vi "Send.vi"(5 "Record Topic Name?":bool, 7 "Message Priority":T1, 8 "error in (no error)":errorcluster, 9 "Timeout":i32, 10 "Message":refnum<class "Message Interface.lvclass">, 11 "Message Transport Queue in":refnum<class "Message Transport Queue.lvclass">) -> (0 "error out":errorcluster, 2 "Timed Out?":bool, 3 "Message Transport Queue out":refnum<class "Message Transport Queue.lvclass">)   [LabVIEW 2016, in "Stream Mediator.lvlib" / "Message Transport Queue.lvclass"]
doc: "--\nCopyright © 2017 Composed SystemsI All rights reserved.\n\nAuthor: Jon McBee <jon.mcbee@composed.io>\n\nThis library is provided \"AS IS\" ,WITHOUT WARRANTIES OR\nCONDITIONS OF ANY KIND, either express or implied.\n\nComposed Systems -- composed.io\n\nStream 0.0.1.1\nJon McBee - Composed Systems\nCopyright (c) 2017, Composed Systems"
uses:
  <userlib>/Composed Systems/Stream/Mediator/Classes/Message Transport Queue/Message Transport Queue.lvclass
  C:/Program Files (x86)/National Instruments/LabVIEW 2016/user.lib/Composed Systems/Stream/Mediator/Classes/Message Transport Interface/Message Transport Interface.lvclass
  <userlib>/Composed Systems/Stream/Mediator/Classes/Message Interface/Message Interface.lvclass
  <userlib>/Composed Systems/Stream/Mediator/Classes/Message Transport Interface/Message Priority.ctl
  <userlib>/Composed Systems/Stream/Mediator/Classes/Message Interface/Message Interface.lvclass/Message Interface.ctl
  <userlib>/Composed Systems/Stream/Mediator/Classes/Message Transport Queue/Message Transport Queue.lvclass/Message Transport Queue.ctl
  <userlib>/Composed Systems/Stream/Mediator/Classes/Message Transport Interface/Message Transport Interface.lvclass
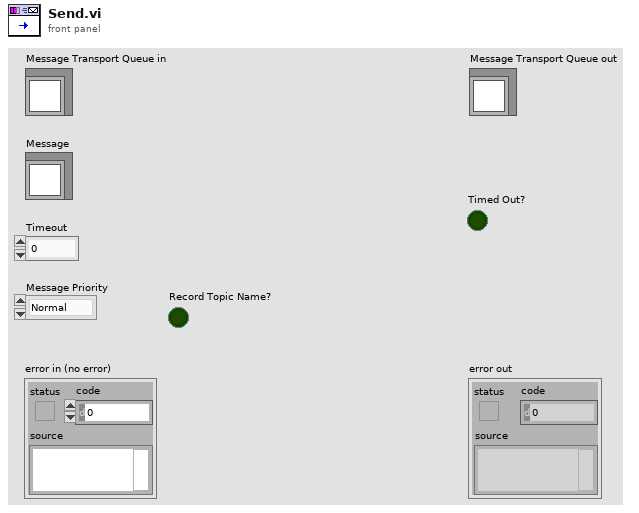
[diagram p1: front panel]
types:
  T1 = typedef "Stream Mediator.lvlib/Message Transport Interface.lvclass/Message Priority.ctl" = enum16{"Normal", "High"}
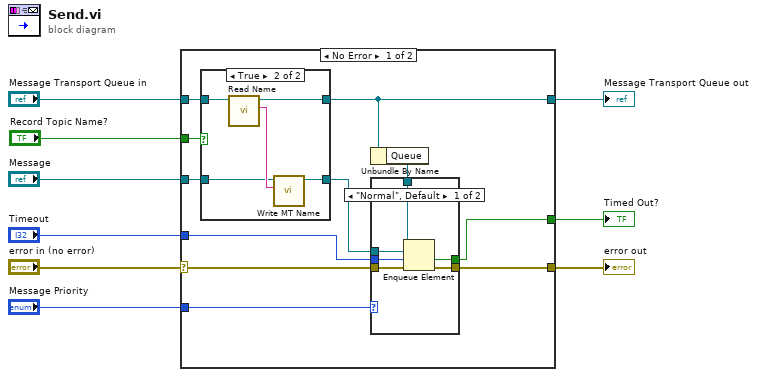
[diagram p0: block diagram]
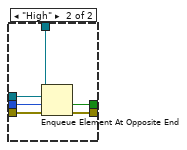
[diagram p3: hidden frame]
diagram:
  n1 = case shown="No Error" "error in (no error)" {
    selector: "error in (no error)" -> [w20 w40]
    tunnel: [w19 w40] -> w8
    tunnel: [w13 w41] -> w7
    tunnel: "Message Transport Queue in" -> [w14 w41]
    tunnel: "Message" -> [w12 _]
    tunnel: "Timeout" -> [w17 _]
    tunnel: "Message Priority" -> [w16 _]
    tunnel: [w15 _] -> w2
    tunnel: "Record Topic Name?" -> [w10 _]
    frame No Error {
      n2 = case shown="True" w10 {
        tunnel: w14 -> [w22 w26]
        tunnel: [w22 w25] -> w13
        tunnel: w12 -> [w21 w24]
        tunnel: [w21 w23] -> w11
        frame False {
        }
        frame True {
          n3 = call <userlib>:"Read Name.vi"("Message Transport Interface in"=w26) -> ("Name"=w27:string, "Message Transport Interface out"=w25:refnum<class "Message Transport Queue.lvclass">)  [unwired: 8 in, 1 out]
          n4 = call <userlib>:"Write MT Name.vi"("MT Name"=w27, "Message Interface in"=w24) -> ("Message Interface out"=w23:refnum<class "Message Interface.lvclass">)  [unwired: 9 in]
        }
      }
      n5 = Unbundle By Name(w13) -> ("Queue"=w18:refnum<queue>)
      n6 = case shown="\"Normal\", Default" w16 {
        tunnel: w20 -> [w33 w39]
        tunnel: [w32 w38] -> w19
        tunnel: w18 -> [w31 w37]
        tunnel: w11 -> [w30 w36]
        tunnel: w17 -> [w29 w35]
        tunnel: [w28 w34] -> w15
        frame "Normal", Default {
          n7 = Enqueue Element(queue=w31, element=w30, timeout in ms (-1)=w29, error in (no error)=w33) -> (timed out?=w28:bool, error out=w32:errorcluster)  [unwired: 1 out]
        }
        frame "High" {
          n8 = Enqueue Element At Opposite End(queue=w37, element=w36, timeout in ms (-1)=w35, error in (no error)=w39) -> (timed out?=w34:bool, error out=w38:errorcluster)  [unwired: 1 out]
        }
      }
    }
    frame Error {
    }
  }
  "error out" <- w8
  "Message Transport Queue out" <- w7
  "Timed Out?" <- w2
